vi "Wrap Calibration Results in Data.vi"(8 "error in (no error)":errorcluster, 10 "Calibration Result":variant, 11 "Calibrate Instrument Msg in":refnum<class "Calibrate Instrument Msg.lvclass">) -> (0 "error out":errorcluster, 2 "Data":refnum<class "Data.lvclass">, 3 "Calibrate Instrument Msg out":refnum<class "Calibrate Instrument Msg.lvclass">)   [LabVIEW 2020, in "Instrument Handler.lvlib" / "Calibrate Instrument Msg.lvclass"]
doc: "Wrap the calibration results in a Data class. If the Variant contains Instrument Data this will be returned, if not a generic Variant class will be returned."
uses:
  Calibrate Instrument Msg.lvclass
  PPL/HDH.Data.Generic.lvlibp/Data.lvclass
  Data/Instrument Data/Instrument Data.lvclass
  C:/Current projects/WS/PPL/HDH.Data.Generic.lvlibp/Data.lvclass
  PPL/HDH.Data.Generic.lvlibp/Generic Data/Variant/Variant.lvclass
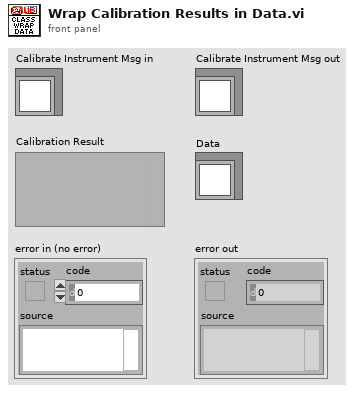
[diagram p1: front panel]
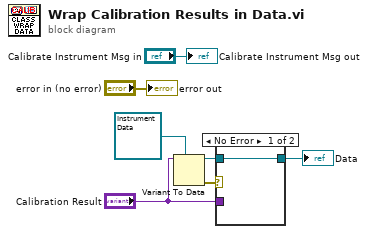
[diagram p0: block diagram]
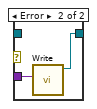
[diagram p2: hidden frame]
diagram:
  n1 = Variant To Data(type=refnum<class "Instrument Data.lvclass"> refnum ("Data"), Variant="Calibration Result") -> (data=w2:refnum<class "Instrument Data.lvclass">, error out=w3:errorcluster)  [unwired: 1 in]
  n2 = case shown="No Error" w3 {
    tunnel: [w8 w9] -> w6
    tunnel: w2 -> [w8 _]
    tunnel: "Calibration Result" -> [_ w10]
    frame No Error {
    }
    frame Error {
      n3 = call "Write.vi"("Variant"=w10) -> ("Variant out"=w9:refnum<class "Variant.lvclass">)  [unwired: 10 in]
    }
  }
  "Data" <- w6
  "error out" <- "error in (no error)"
  "Calibrate Instrument Msg out" <- "Calibrate Instrument Msg in"
